vi "Lockin_Amplifier_diag_optional.vi"(0 "Reference signal (dialog if empty)":path=path "D:/#Meresek/Malaria/Malaria_measurement_program/Labview/Lock_in_Amplifier/tesztsor/timetrace_46.txt", 1 "Sample Number":i32=100000, 2 "DC(V)":dbl, 3 "Cutoff Frequency":dbl=500.0, 4 "dt":dbl=0.0002, 5 "Window (s)":dbl=3.0, 6 "Continous Lock-in":bool, 7 "Resolution":dbl=0.0001, 8 "averaging time":dbl=1.0 format="%0.2p", 9 "Error In":errorcluster, 11 "Second":bool, 12 "Sampling Freq":dbl=5000.0, 14 "tolerance (Deviation)":dbl=3.0) -> (13 "Error Out":errorcluster, 15 "dLD_RMS":dbl, 16 "LD_RMS":dbl, 17 "Signal Spectrum":cluster{"f0":dbl, "df":dbl, "magnitude":dbl[]}[](graph), 18 "LockIN R (cont/disc)":waveform(dbl)(graph), 19 "MLD & Phase":T1, 23 "Time Domain Signal":cluster{"xi used":dbl[], "yi":dbl[]}[](graph), 24 "Phase average":dbl format="%0.2f", 25 "Phase  deviation":dbl format="%0.2f", 26 "Timetrace_ref":waveform(dbl)[](array[waveform]), 27 "LockIN Theta (cont/disc)":waveform(dbl)(graph))   [LabVIEW 2013]
uses:
  <vilib>/Utility/file.llb/Read From Spreadsheet File (DBL).vi
  <vilib>/gmath/NI_Gmath.lvlib
panel:
  out "Averaging window":dbl
  in  "Tab Control":T2(tab)
  out "Reference signal / PLL Signal":cluster{"all rows":dbl[], "all rows":dbl[]}[](graph)
  out "Reference Spectrum":cluster{"f0":dbl, "df":dbl, "magnitude":dbl[]}(graph)
  out "Synthetized Spectrum":cluster{"f0":dbl, "df":dbl, "magnitude":dbl[]}(graph)
  in  "t0_ref":dbl
  in  "t0_LD":dbl=0.0001
  out "LD Spectrum (Vrms)":cluster{"f0":dbl, "df":dbl, "magnitude":dbl[]}(graph)
  out "Tolerance Level":dbl
  out "average":dbl
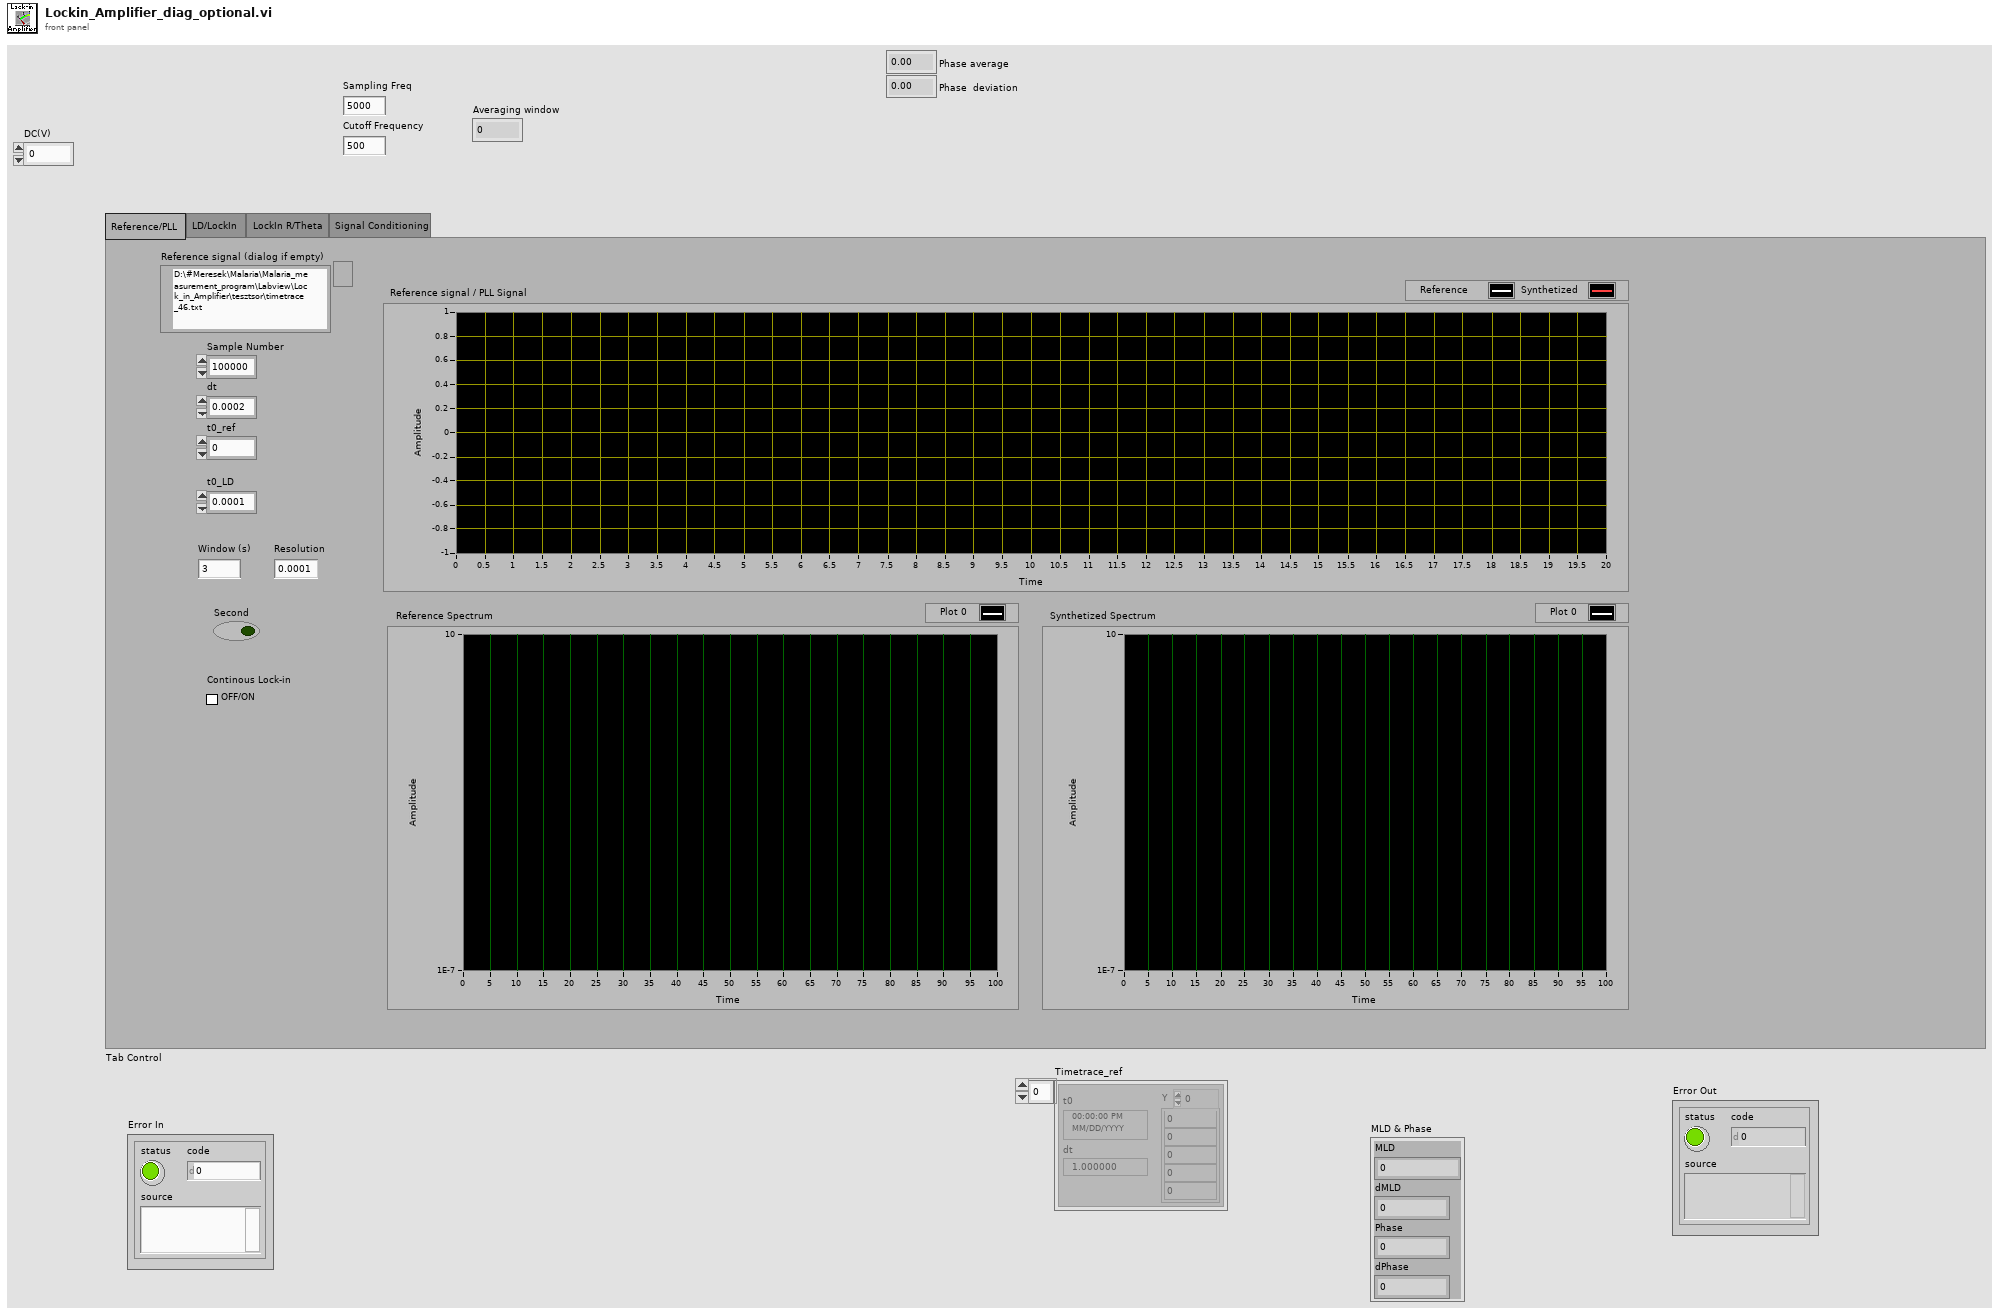
[diagram p1: front panel]
types:
  T1 = cluster{"MLD":dbl, "dMLD":dbl, "Phase":dbl, "dPhase":dbl}
  T2 = enum32{"Reference/PLL", "LD/LockIn", "LockIn R/Theta", "Signal Conditioning"}
  T3 = cluster{"Lockin R":dbl, "dR":dbl, "dTheta":dbl, "Theta":dbl}
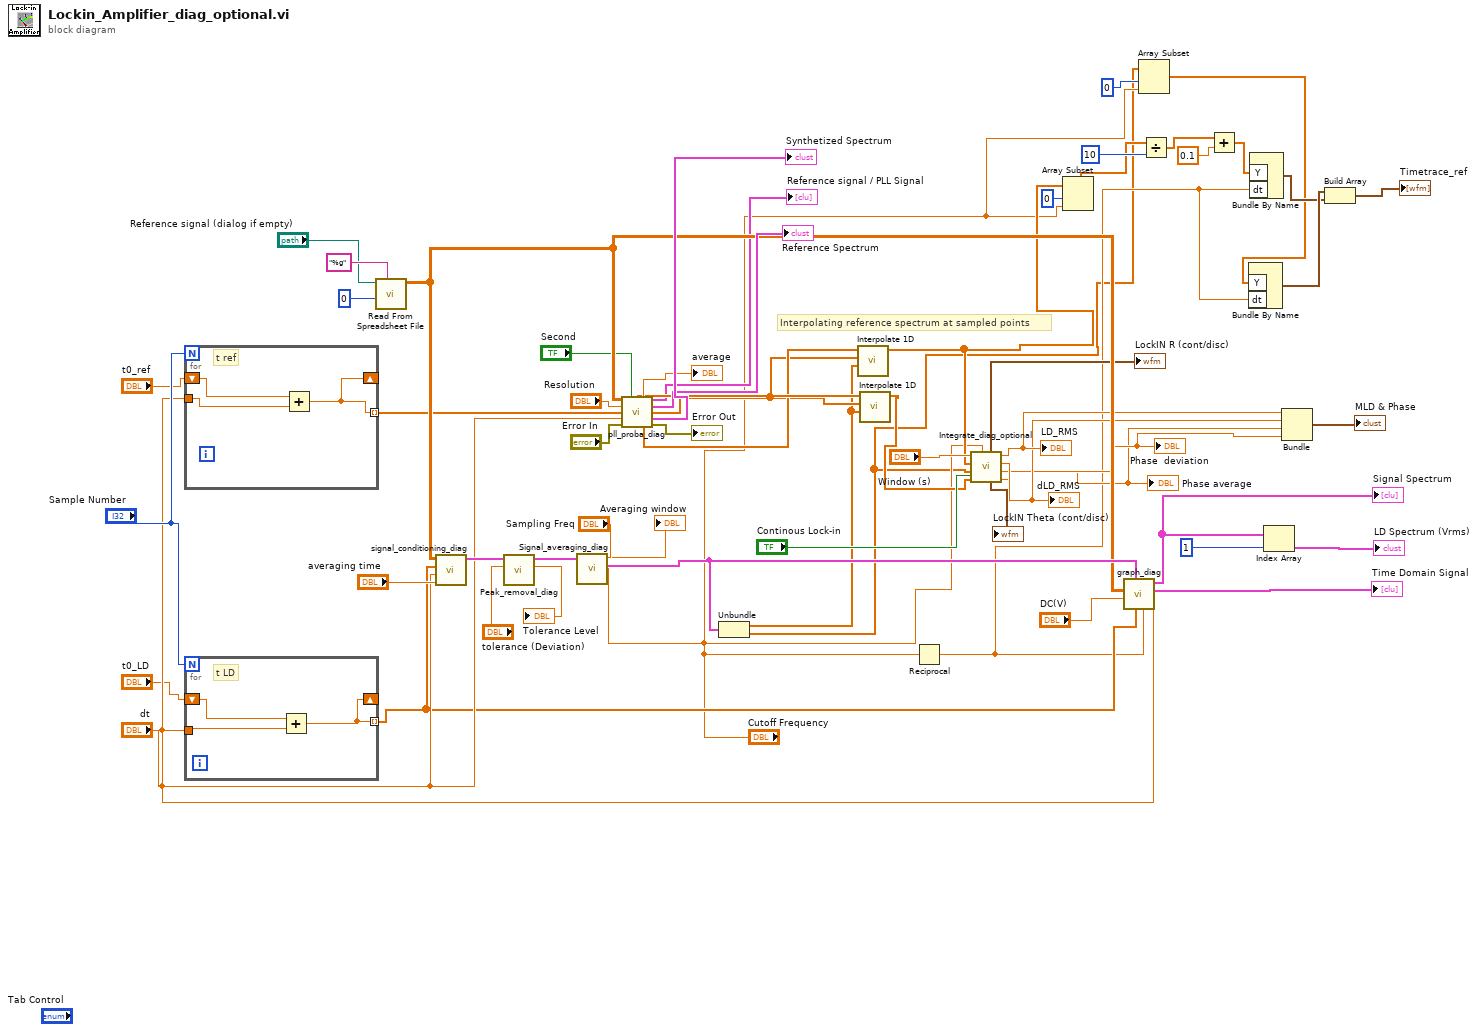
[diagram p0: block diagram]
diagram:
  # "Interpolating reference spectrum at sampled points"
  n1 = for {
    N: "Sample Number" -> [_]
    tunnel: "dt" -> [w62]
    tunnel: [w61] -> w20 mode=indexing
    shift-right: [w61] -> _
    shift-left: "t0_ref" -> [w63]
    # "t ref"
    n2 = Add(x=w63, y=w62) -> (x+y=w61:dbl)
  }
  n3 = for {
    N: "Sample Number" -> [_]
    shift-right: [w65] -> _
    shift-left: "t0_LD" -> [w66]
    tunnel: "dt" -> [w64]
    tunnel: [w65] -> w17 mode=indexing
    # "t LD"
    n4 = Add(x=w66, y=w64) -> (x+y=w65:dbl)
  }
  n5 = call-poly <vilib>:"Read From Spreadsheet File.vi"("format (%.3f)"="%g" ("format (%.6f)"), "start of read offset (chars.:0)"=0, "file path (dialog if empty)"="Reference signal (dialog if empty)") -> ("all rows"=w35:dbl[][])  [unwired: 4 in, 4 out]
  n6 = call "signal_conditioning_diag.vi"("averaging time"="averaging time", "dt"="dt", "t_LD"=w17, "all rows"=w35) -> ("Offset removed"=w47:cluster{"xi used":dbl[], "yi":dbl[]})  [unwired: 6 in, 1 out]
  n7 = call "Peak_removal_diag.vi"("tolerance (Deviation)"="tolerance (Deviation)", "Offset removed"=w47) -> ("Tolerance Level"=→"Tolerance Level":dbl, "XY Graph"=w44:cluster{"xi used":dbl[], "yi":dbl[]})  [unwired: 8 in]
  n8 = call "Signal_averaging_diag.vi"("Pike removed"=w44, "Cutoff Frequency"="Cutoff Frequency", "Sampling Freq"="Sampling Freq") -> ("Averaged"=w43:cluster{"xi used":dbl[], "yi":dbl[]}, "Averaging window"=→"Averaging window":dbl)  [unwired: 7 in]
  n9 = call "pll_proba_diag.vi"("all rows"=w35, "Second"="Second", "Resolution"="Resolution", "t_ref"=w20, "dt"="dt", "Error In"="Error In") -> ("average"=→"average":dbl, "XY Graph"=→"Reference signal / PLL Signal":cluster{"all rows":dbl[], "all rows":dbl[]}[], "Waveform Graph"=→"Reference Spectrum":cluster{"f0":dbl, "df":dbl, "magnitude":dbl[]}, "time"=w51:dbl[], "Waveform Graph 2"=→"Synthetized Spectrum":cluster{"f0":dbl, "df":dbl, "magnitude":dbl[]}, "PLL_sine"=w53:dbl[], "PLL_cosine"=w52:dbl[], "Error Out"=→"Error Out":errorcluster)  [unwired: 2 in]
  n10 = Unbundle(w43) -> ("xi used"=w28:dbl[], "yi"=w2:dbl[])
  n11 = call <vilib>:"Interpolate 1D.vi"("xi"=w28, "X"=w51, "Y"=w52) -> ("yi"=w7:dbl[])  [unwired: 6 in, 2 out]
  n12 = call <vilib>:"Interpolate 1D.vi"("xi"=w28, "X"=w51, "Y"=w53) -> ("yi"=w29:dbl[])  [unwired: 6 in, 2 out]
  n13 = Reciprocal(x="Cutoff Frequency") -> (1/x=w15:dbl)
  n14 = call "Integrate_diag_optional.vi"("Continous Lock-in"="Continous Lock-in", "Cutoff Frequency"="Cutoff Frequency", "Ref Sine"=w29, "Processed LD values"=w2, "Ref Cosine"=w7, "Window (s)"="Window (s)") -> ("dTheta"=w22:dbl, "Theta"=w23:dbl, "dR"=w24:dbl, "Lockin R"=w25:dbl, "Phase (deg)"=→"LockIN Theta (cont/disc)":waveform(dbl), "LockIN R (cont/disc)"=→"LockIN R (cont/disc)":waveform(dbl))
  "LD_RMS" <- w25
  "dLD_RMS" <- w24
  "Phase average" <- w22
  "Phase  deviation" <- w23
  n15 = Array Subset(array=w7, index=0, length="Cutoff Frequency") -> (w6:dbl[])
  n16 = call "graph_diag.vi"(4:"dt"=w15, "Array in"=w17, "Averaged"=w43, "DC(V)"="DC(V)", "LD Timetrace in"=w35, 11:"dt"="dt") -> ("Time Domain Signal"=→"Time Domain Signal":cluster{"xi used":dbl[], "yi":dbl[]}[], "Spectra"=w39:cluster{"f0":dbl, "df":dbl, "magnitude":dbl[]}[])  [unwired: 4 in]
  "Signal Spectrum" <- w39
  n17 = Array Subset(array=w2, index=0, length="Cutoff Frequency") -> (w1:dbl[])
  n18 = Divide(x=w6, y=10) -> (x/y=w10:dbl[])
  n19 = Add(x=w10, y=0.1) -> (x+y=w8:dbl[])
  n20 = Bundle By Name("Y"=w1, "dt"=w15) -> (w14:waveform(dbl))  [unwired: 1 in]
  n21 = Bundle By Name("Y"=w8, "dt"=w15) -> (w13:waveform(dbl))  [unwired: 1 in]
  n22 = Index Array(array=w39, index=1) -> (element=→"LD Spectrum (Vrms)":cluster{"f0":dbl, "df":dbl, "magnitude":dbl[]})
  n23 = Bundle("Lockin R"=w25, "dR"=w24, "dTheta"=w22, "Theta"=w23) -> (→"MLD & Phase":T3)  [unwired: 1 in]
  n24 = Build Array(w14, w13) -> (→"Timetrace_ref":waveform(dbl)[])
